vi "Shutdown.vi"(8 "error in (no error)":errorcluster, 11 "Modbus master in":refnum<class "Modbus Master.lvclass">) -> (0 "error out":errorcluster)   [LabVIEW 2021, in "Modbus Master.lvclass"]
doc: "Closes and destroys a Modbus master instance."
uses:
  Modbus Master.lvclass
  D:/my_projects/projects/Algorithms/Labview/21/Modbus_v121c/API/Modbus API.lvclass
  Modbus API.lvclass/Modbus API.ctl
  Read Network Protocol.vi
  Network Protocol/Network Master/Network Master.lvclass
  D:/my_projects/projects/Algorithms/Labview/21/Modbus_v121c/Network Protocol/Network Protocol.lvclass
  Modbus Master.lvclass/Modbus Master.ctl
  Modbus API.lvclass
panel:
  out "Modbus master OUT":refnum<class "Modbus Master.lvclass">
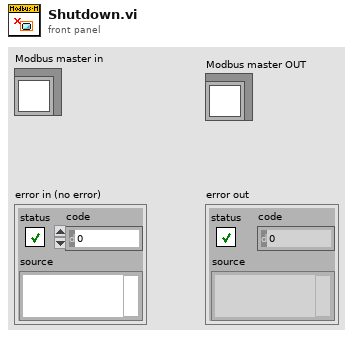
[diagram p1: front panel]
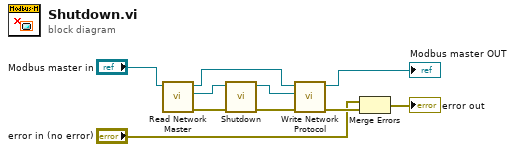
[diagram p0: block diagram]
diagram:
  n1 = call "Read Network Master.vi"("Modbus master in"="Modbus master in") -> ("error out"=w1:errorcluster, "Network Master"=w2:refnum<class "Network Master.lvclass">, "Modbus master out"=w5:refnum<class "Modbus Master.lvclass">)  [unwired: 8 in]
  n2 = call-dynamic "Shutdown.vi"("error in"=w1, "Network Master in"=w2) -> ("error out"=w7:errorcluster, "Network Master out"=w8:refnum<class "Network Master.lvclass">)  [unwired: 8 in]
  n3 = call "Write Network Protocol.vi"("error in (no error)"=w7, "Network Protocol"=w8, "Modbus API in"=w5) -> ("error out"=w9:errorcluster, "Modbus API out"=→"Modbus master OUT":refnum<class "Modbus Master.lvclass">)  [unwired: 7 in]
  n4 = Merge Errors("error in (no error)", w9) -> (→"error out":errorcluster)
